vi "getAbsInt.vi"(4 "Fiber Num":i32, 6 "Error":bool, 7 "VISA resource name":refnum<visa-resource-name>="ASRL13::INSTR") -> (0 "Absolute Intensity":dbl, 2 "Error":bool, 3 "dup VISA resource name":refnum<visa-resource-name>="ASRL13::INSTR")   [LabVIEW 2018]
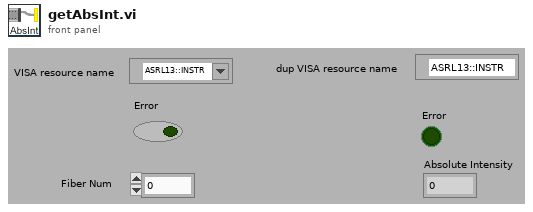
[diagram p1: front panel]
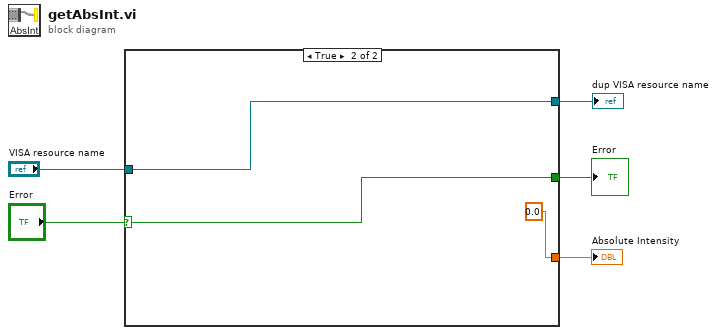
[diagram p0: block diagram]
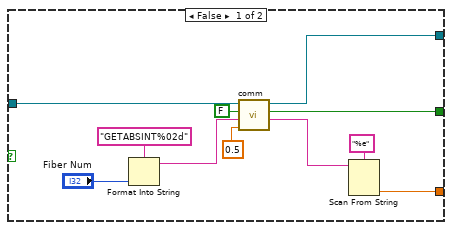
[diagram p2: hidden frame]
diagram:
  n1 = case shown="True" "Error" {
    selector: "Error" -> [_ w18]
    tunnel: "VISA resource name" -> [w16 w19]
    tunnel: [w10 0.0] -> w4
    tunnel: [w6 w19] -> w2
    tunnel: [w7 w18] -> w1
    frame False {
      n2 = Format Into String(format string="GETABSINT%02d" ("Substring"), "Fiber Num") -> (resulting string=w13:string)  [unwired: 2 in, 1 out]
      n3 = call "comm.vi"("Timeout (s)"=0.5, "Command"=w13, "Error"=FALSE, "VISA resource name"=w16) -> ("Response"=w12:string, "Error"=w7:bool, "dup VISA resource name"=w6:refnum<visa-resource-name>)  [unwired: 2 in, 1 out]
      n4 = Scan From String(format string="%e", input string=w12) -> (output 1=w10:dbl)  [unwired: 3 in, 3 out]
    }
    frame True {
    }
  }
  "Absolute Intensity" <- w4
  "Error" <- w1
  "dup VISA resource name" <- w2
